vi "Drive Controller.vi"(8 "error in":errorcluster) -> ()   [LabVIEW 2017]
doc: "This VI executes continuously carrying out the current operation and responding to updates or new operation requests. It will often contain the timing or control code that is difficult to place directly in TeleOp. This VI generally opens all sensors and motors and isolates the rest of the robot code from knowing implementation details of how the operations are carried out."
uses:
  <vilib>/Rock Robotics/WPI/Framework/Completion Status.ctl
  Drive Setpoints.ctl
  Drive Operations.ctl
  Shared/RobotNeededPathData.ctl
  <vilib>/Rock Robotics/SystemInterfaces/DIO/FPGA_DIOPWMChannel.ctl
  <vilib>/Rock Robotics/WPI/SafetyOutput/WPI_SafetyOutputConfigMenu.ctl
  <vilib>/Rock Robotics/SystemInterfaces/DIO/FPGA_DIOChannel.ctl
  <vilib>/Rock Robotics/WPI/DriverStation/WPI_DriverStationRobotMode2.ctl
  <vilib>/Rock Robotics/WPI/RobotDrive/WPI_RobotDriveOpen2MotorWithSPARK.vi
  <vilib>/Rock Robotics/WPI/RobotDrive/WPI_RobotDriveOpen4MotorWithSPARK.vi
  <vilib>/Rock Robotics/WPI/Counter/WPI_CounterDigitalInputToDigitalSource.vi
  <vilib>/Rock Robotics/Network Tables/NT Read Number.vi
  Drive Published Globals.vi
  Framework/Robot Global Data.vi
  Configuration/Constants.vi
  <vilib>/Rock Robotics/WPI/ThirdParty/Sensors/navX/_Processing Loop/FRIC_navX_Internal_SPI_ProcessingLoop.vi
panel:
  in  "LookAhead":dbl=15.0 format="%#_13g"
  in  "Trackwidth":dbl=40.0 format="%#_13g"
  out "Yaw":dbl
  in  "Zero Yaw":bool
  in  "Gains":T1={"FFV"=0.0088, "FFA"=0.0017, "Vel PID"={"P"=0.01, "I"=0.007, "D"=0.0}}
  in  "Interactive Values":T2
  in  "Buttons":cluster{"Execute Cmd":bool, "Abort Cmd":bool}
  out "Command Timing":cluster{"Start Time (ms)":u32, "Iterations":i32}
  out "Status":T5
  out "Setpoints":T6(graph)
  out "Current\nCmd":string
  # "Tip: The graph shows the motor setpoints. It may also be helpful to observe inputs and sensor values.\nYou may also want to display tuning or debugging controls."
  # "Interactive Command: You may fill in the settings for a command\nand schedule it with the Execute button. You can observe and abort\nany command while fine tuning the code for the controller."
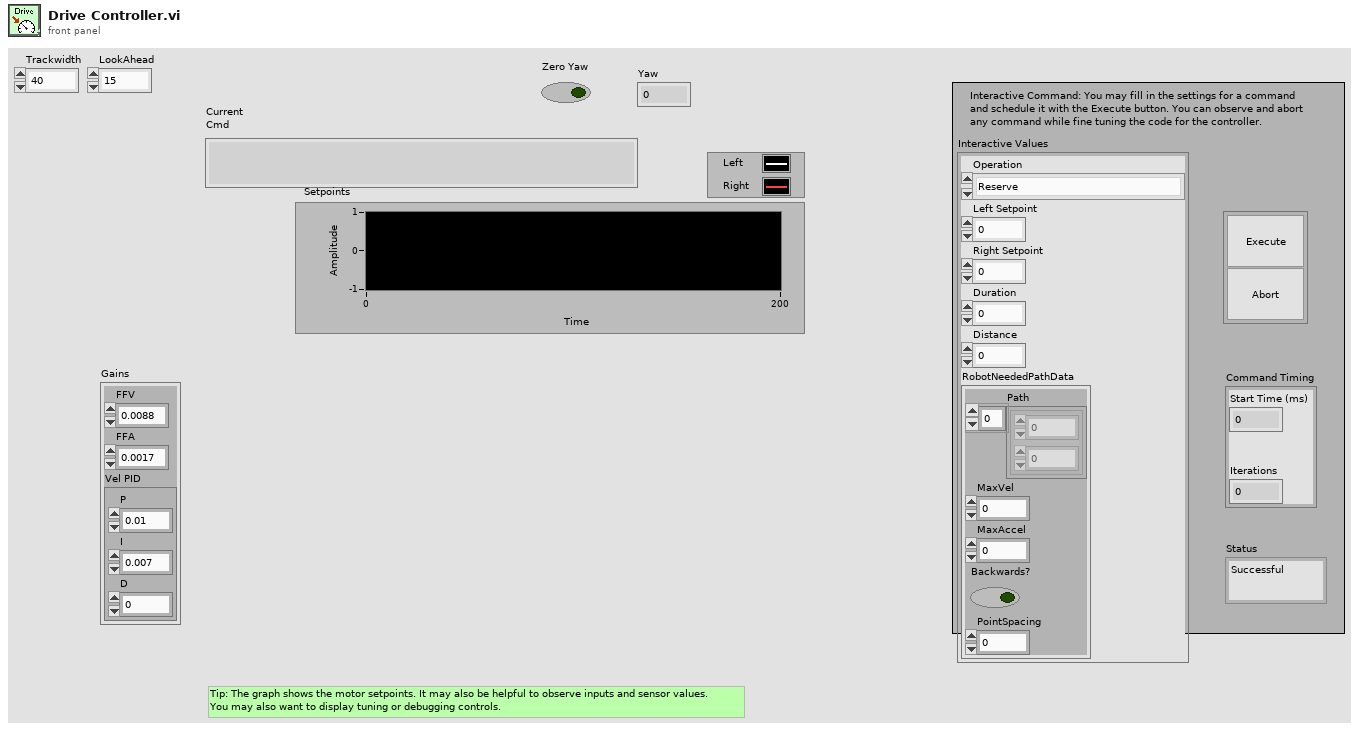
[diagram p1: front panel]
types:
  T1 = cluster{"FFV":dbl, "FFA":dbl, "Vel PID":cluster{"P":dbl, "I":dbl, "D":dbl}}
  T2 = typedef "Drive Setpoints.ctl" = cluster{"Operation":T3, "Left Setpoint":dbl, "Right Setpoint":dbl, "Duration":dbl, "Distance":dbl, "RobotNeededPathData":T4}
  T3 = typedef "Drive Operations.ctl" = enum16{"Reserve", "Read Current", "Immediate", "Drive for Time", "Drive for Distance", "Drive Path"}
  T4 = typedef "RobotNeededPathData.ctl" = cluster{"Path":cluster{dbl, dbl}[], "MaxVel":dbl, "MaxAccel":dbl, "Backwards?":bool, "PointSpacing":dbl}
  T5 = typedef "Completion Status.ctl" = enum16{"Successful", "Aborted", "Incomplete"}
  T6 = cluster{"Left Setpoint":dbl, "Right Setpoint":dbl}
  T7 = typedef "FPGA_DIOChannel.ctl" = enum8{"DIO 0", "DIO 1", "DIO 2", "DIO 3", "DIO 4", "DIO 5", "DIO 6", "DIO 7", "DIO 8", "DIO 9", "DIO MXP 0", "DIO MXP 1", "DIO MXP 2", "DIO MXP 3", "DIO MXP 4", "DIO MXP 5", "DIO MXP 6", "DIO MXP 7", "DIO MXP 8", "DIO MXP 9", "DIO MXP 10", "DIO MXP 11", "DIO MXP 12", "DIO MXP 13", "DIO MXP 14", "DIO MXP 15", "SPI Port CS1", "SPI Port CS2", "SPI Port CS3", "SPI Port MISO", "SPI Port MOSI", "Invalid"}
  T8 = typedef "WPI_SafetyOutputConfigMenu.ctl" = enum16{"Enable", "Disable"}
  T9 = typedef "FPGA_DIOPWMChannel.ctl" = enum8{"PWM 0", "PWM 1", "PWM 2", "PWM 3", "PWM 4", "PWM 5", "PWM 6", "PWM 7", "PWM 8", "PWM 9", "PWM MXP 0", "PWM MXP 1", "PWM MXP 2", "PWM MXP 3", "PWM MXP 4", "PWM MXP 5", "PWM MXP 6", "PWM MXP 7", "PWM MXP 8", "PWM MXP 9", "Invalid"}
  T10 = typedef "WPI_DigitalInputDevRef.ctl" = cluster{"DevStatus":errorcluster, "DIO Channel":T7}
  T11 = typedef "FPGA_CounterEncoderSourceConvertionLVSourceType.ctl" = cluster{"DevStatus":errorcluster, "AnalogTriggerMode?":bool, "DigitalMode":cluster{"DIO Channel":T12}, "AnalogTriggerMode":cluster{"AnalogTriggerIndex":T13, "OutputType":T14}}
  T12 = typedef "FPGA_DIODigitalSourceChannel.ctl" = enum8{"DIO 0", "DIO 1", "DIO 2", "DIO 3", "DIO 4", "DIO 5", "DIO 6", "DIO 7", "DIO 8", "DIO 9", "DIO MXP 0", "DIO MXP 1", "DIO MXP 2", "DIO MXP 3", "DIO MXP 4", "DIO MXP 5", "DIO MXP 6", "DIO MXP 7", "DIO MXP 8", "DIO MXP 9", "DIO MXP 10", "DIO MXP 11", "DIO MXP 12", "DIO MXP 13", "DIO MXP 14", "DIO MXP 15", "Disabled"}
  T13 = typedef "FPGA_AnalogTriggerIndex.ctl" = enum8{"Trig 0", "Trig 1", "Trig 2", "Trig 3", "Trig 4", "Trig 5", "Trig 6", "Trig 7", "Invalid"}
  T14 = typedef "FPGA_AnalogTriggerOutType.ctl" = enum16{"InWindow", "TriggerState", "Rising", "Falling"}
  T15 = typedef "WPI_EncoderDevRef.ctl" = cluster{"DevStatus":errorcluster, "EncoderIndex":T16, "CounterIndex":T17, "DistancePerCount":dbl, "Decoding Type":T18}
  T16 = typedef "FPGA_EncoderIdx.ctl" = enum8{"Enc 0", "Enc 1", "Enc 2", "Enc 3", "Enc 4", "Enc 5", "Enc 6", "Enc 7", "Invalid"}
  T17 = typedef "FPGA_CounterCtrSystemIndex.ctl" = enum8{"Ctr 0", "Ctr 1", "Ctr 2", "Ctr 3", "Ctr 4", "Ctr 5", "Ctr 6", "Ctr 7", "Invalid"}
  T18 = typedef "WPI_EncoderType.ctl" = enum16{"1x", "2x", "4x"}
  T19 = typedef "WPI_RobotDriveDevRef.ctl" = cluster{"DevStatus":errorcluster, "Motors[]":T20[], "Square Inputs":bool, "Max Output":dbl}
  T20 = typedef "WPI_MotorControlDeviceRef.ctl" = cluster{"DeviceStatus":errorcluster, "Type":T21, "PWM":cluster{"PWM Channel":T9, "DeadBand":T22}, "CAN":cluster{"Device Number":u8, "SetOutput VI Ref":variant, "GetOutput VI Ref":variant, "Enable VI Ref":variant, "Disable VI Ref":variant, "Data":variant}, "Invert":bool, "DIO PWM":cluster{"PWM \"Enable\" Channel":T9, "DIOChannel":T7, "PWM Rate":dbl}}
  T21 = typedef "WPI_MotorControlType.ctl" = enum16{"PWM", "CAN", "DIO PWM"}
  T22 = typedef "WPI_PWMDeadband.ctl" = cluster{"Name":string, "maxPositivePwm":i32, "minPositivePwm":i32, "centerPwm":i32, "maxNegativePwm":i32, "minNegativePwm":i32, "angularRange":u16}
  T23 = cluster{"RobotDriveDevRef":T19, "RobotDriveDevRef":T19}
  T24 = typedef "Command Status Info.ctl" = cluster{"Name":string, "Status":T5, "notifier out":T25}
  T25 = typedef "Completion Notifier.ctl" = refnum<notifier>
  T26 = cluster{"SubSystem Data":T2, cluster{"Start Time (ms)":u32, "Iterations":i32}, cluster{"Command Info":T24, "Description":string, "Default Command":T2, "queue out":refnum<queue>, "Subsystem Name":string}}
  T27 = cluster{"LeftDistance":dbl, "RightDistance":dbl, "LeftVelocity":dbl, "RightVelocity":dbl, "Angle":dbl, "Location":cluster{dbl, dbl}}
  T28 = cluster{"dx/dt":dbl, "dx/dt":dbl, "Yaw":dbl, cluster{dbl, dbl}}
  T29 = cluster{"Path":cluster{dbl, dbl}[], "PointSpacing":dbl}
  T30 = cluster{"SubSystem Data":T2, cluster{"Start Time (ms)":u32, "Iterations":i32}, "Default Command Arguments":cluster{"Command Info":T24, "Description":string, "Default Command":T2, "queue out":refnum<queue>, "Subsystem Name":string}}
  T31 = typedef "WPI_DriverStationRobotMode2.ctl" = enum16{"Autonomous Disabled", "Autonomous Enabled", "Teleop Disabled", "Teleop Enabled", "Disconnected", "Finish", "Test Disabled", "Test Enabled", "Emergency Stopped"}
  T32 = cluster{"Yaw":dbl, "Roll":dbl, "Pitch":dbl, "Heading":dbl, "Fused Heading":dbl}
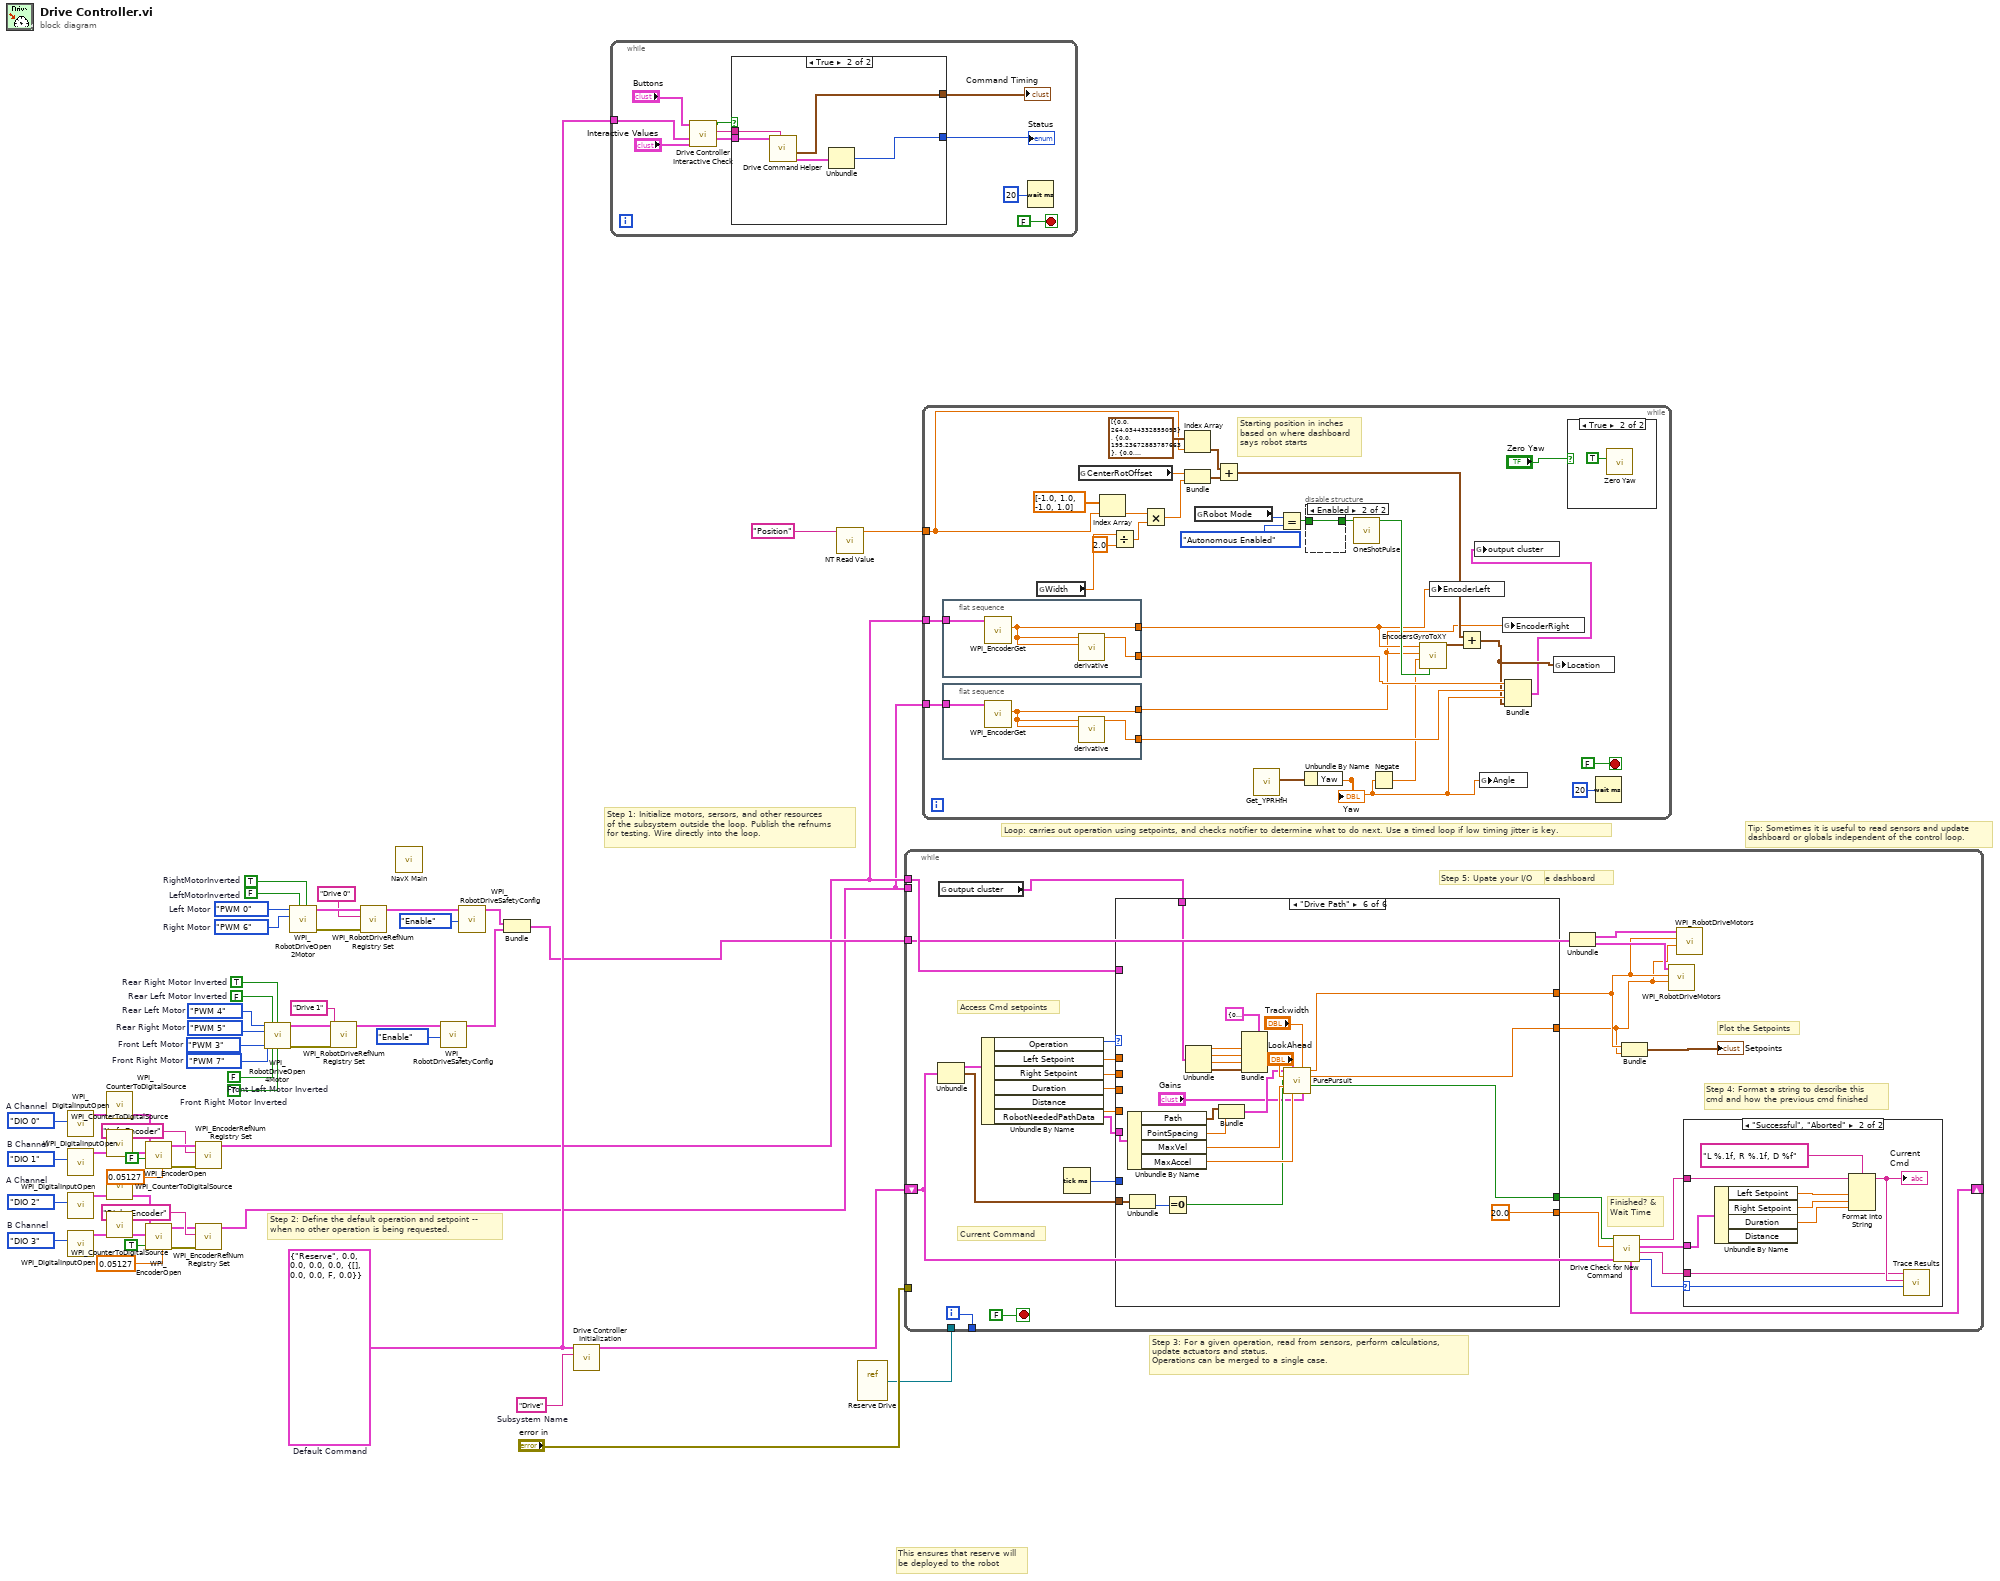
[diagram p0: block diagram]
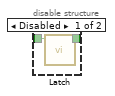
[diagram p2: hidden frame]
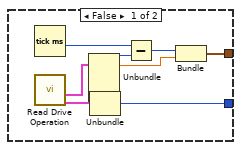
[diagram p4: hidden frame]
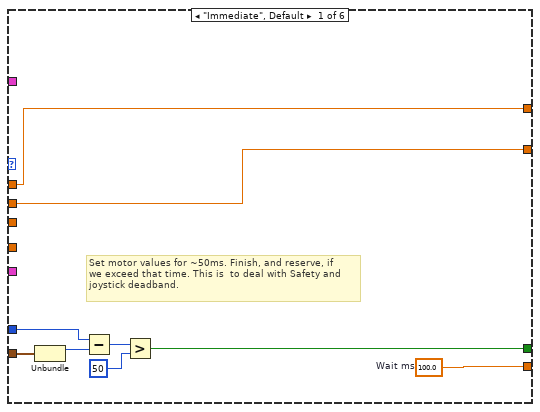
[diagram p5: hidden frame]
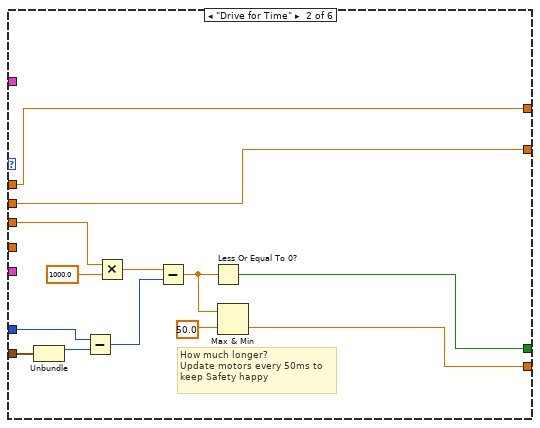
[diagram p6: hidden frame]
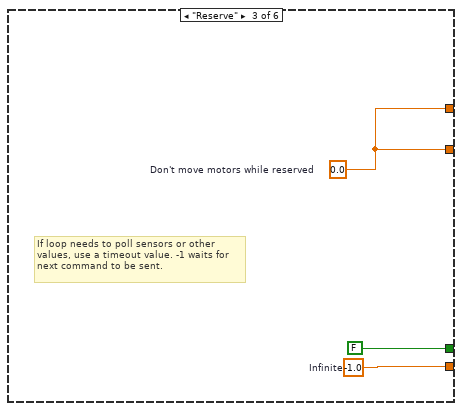
[diagram p7: hidden frame]
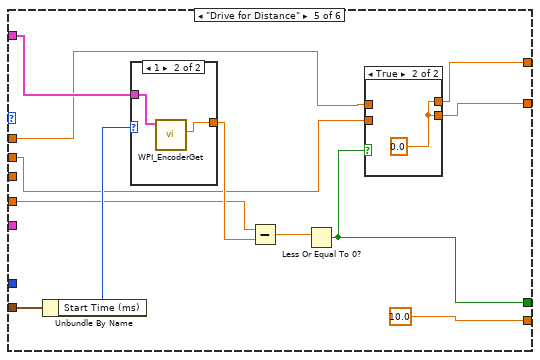
[diagram p9: hidden frame]
diagram:
  w9 = FPGA_DIOChannel."DIO 3"  # B Channel
  w10 = FPGA_DIOChannel."DIO 2"  # A Channel
  w26 = FPGA_DIOChannel."DIO 1"  # B Channel
  w25 = FPGA_DIOChannel."DIO 0"  # A Channel
  w32 = TRUE  # Front Right Motor Inverted
  w33 = FALSE  # Front Left Motor Inverted
  w34 = FALSE  # Rear Left Motor Inverted
  w35 = TRUE  # Rear Right Motor Inverted
  w38 = FPGA_DIOPWMChannel."PWM 7"  # Front Right Motor
  w39 = FPGA_DIOPWMChannel."PWM 3"  # Front Left Motor
  w40 = FPGA_DIOPWMChannel."PWM 5"  # Rear Right Motor
  w41 = FPGA_DIOPWMChannel."PWM 4"  # Rear Left Motor
  w46 = FPGA_DIOPWMChannel."PWM 6"  # Right Motor
  w47 = FPGA_DIOPWMChannel."PWM 0"  # Left Motor
  w50 = FALSE  # LeftMotorInverted
  w51 = TRUE  # RightMotorInverted
  w52 = T2 {"Operation"=enum."Reserve", "Left Setpoint"=0.0, "Right Setpoint"=0.0, "Duration"=0.0, "Distance"=0.0, "RobotNeededPathData"={"Path"=[], "MaxVel"=0.0, "MaxAccel"=0.0, "Backwards?"=FALSE, "PointSpacing"=0.0}}  # Default Command
  w56 = "Drive"  # Subsystem Name
  # "Step 3: For a given operation, read from sensors, perform calculations,\nupdate actuators and status.\nOperations can be merged to a single case."
  # "Step 2: Define the default operation and setpoint --\nwhen no other operation is being requested."
  # "This ensures that reserve will\nbe deployed to the robot"
  # "Tip: Sometimes it is useful to read sensors and update\ndashboard or globals independent of the control loop."
  # "Step 1: Initialize motors, sersors, and other resources\nof the subsystem outside the loop. Publish the refnums\nfor testing. Wire directly into the loop."
  # "Loop: carries out operation using setpoints, and checks notifier to determine what to do next. Use a timed loop if low timing jitter is key."
  n1 = call <vilib>:"WPI_DigitalInputOpen.vi"("DIO Channel"=w25) -> ("DigitalInputDevRef"=w22:T10)  [unwired: 1 in, 9 out]
  n2 = call <vilib>:"WPI_DigitalInputOpen.vi"("DIO Channel"=w26) -> ("DigitalInputDevRef"=w23:T10)  [unwired: 1 in, 9 out]
  n3 = call <vilib>:"WPI_DigitalInputOpen.vi"("DIO Channel"=w10) -> ("DigitalInputDevRef"=w13:T10)  [unwired: 1 in, 9 out]
  n4 = call <vilib>:"WPI_DigitalInputOpen.vi"("DIO Channel"=w9) -> ("DigitalInputDevRef"=w12:T10)  [unwired: 1 in, 9 out]
  n5 = call-poly <vilib>:"WPI_CounterToDigitalSource.vi"("DigitalInputDevRef"=w22) -> ("Digital Source"=w21:T11)  [unwired: 6 out]
  n6 = call-poly <vilib>:"WPI_CounterToDigitalSource.vi"("DigitalInputDevRef"=w23) -> ("Digital Source"=w24:T11)  [unwired: 6 out]
  n7 = call-poly <vilib>:"WPI_CounterToDigitalSource.vi"("DigitalInputDevRef"=w13) -> ("Digital Source"=w14:T11)  [unwired: 6 out]
  n8 = call-poly <vilib>:"WPI_CounterToDigitalSource.vi"("DigitalInputDevRef"=w12) -> ("Digital Source"=w11:T11)  [unwired: 6 out]
  n9 = call <vilib>:"WPI_EncoderOpen.vi"("DistancePerCount"=0.05127, "Invert Direction (False)"=FALSE, "BSource"=w24, "ASource"=w21) -> ("error out"=w20:errorcluster, "EncoderDevRef"=w19:T15)  [unwired: 4 in, 2 out]
  n10 = call <vilib>:"WPI_EncoderOpen.vi"("DistancePerCount"=0.05127, "Invert Direction (False)"=TRUE, "BSource"=w11, "ASource"=w14) -> ("error out"=w15:errorcluster, "EncoderDevRef"=w16:T15)  [unwired: 4 in, 2 out]
  n11 = call <vilib>:"WPI_EncoderRefNum Registry Set.vi"("error in (no error)"=w20, "refnum name"="Left Encoder", "EncoderDevRef"=w19) -> ("EncoderDevRef"=w4:T15)  [unwired: 7 in, 1 out]
  n12 = call <vilib>:"WPI_EncoderRefNum Registry Set.vi"("error in (no error)"=w15, "refnum name"="Right Encoder", "EncoderDevRef"=w16) -> ("EncoderDevRef"=w3:T15)  [unwired: 7 in, 1 out]
  n13 = call-poly <vilib>:"WPI_RobotDriveOpen4Motor.vi"("Rear Left Motor"=w41, "Rear Left Motor Inverted"=w34, "Rear Right Motor Inverted"=w35, "Rear Right Motor"=w40, "Front Left Motor"=w39, "Front Right Motor"=w38, "Front Left Motor Inverted"=w33, "Front Right Motor Inverted"=w32) -> ("RobotDriveDevRef"=w42:T19, "error out"=w43:errorcluster)  [unwired: 6 in]
  n14 = call-poly <vilib>:"WPI_RobotDriveOpen2Motor.vi"("Right Motor Inverted"=w51, "Left Motor Inverted"=w50, "Right Motor"=w46, "Left Motor"=w47) -> ("error out"=w48:errorcluster, "RobotDriveDevRef"=w49:T19)  [unwired: 1 in, 5 out]
  n15 = call <vilib>:"WPI_RobotDriveRefNum Registry Set.vi"("error in (no error)"=w43, "refnum name"="Drive 1", "RobotDriveDevRef"=w42) -> ("RobotDriveDevRef"=w37:T19)  [unwired: 7 in, 1 out]
  n16 = call <vilib>:"WPI_RobotDriveRefNum Registry Set.vi"("error in (no error)"=w48, "refnum name"="Drive 0", "RobotDriveDevRef"=w49) -> ("RobotDriveDevRef"=w45:T19)  [unwired: 1 in, 7 out]
  n17 = call-poly <vilib>:"NavX Main.vi"() -> ()  [unwired: 12 in]
  n18 = call <vilib>:"WPI_RobotDriveSafetyConfig.vi"("mode"=WPI_SafetyOutputConfigMenu."Enable", "RobotDriveDevRef"=w37) -> ("RobotDriveDevRef"=w28:T19)  [unwired: 8 in, 1 out]
  n19 = call <vilib>:"WPI_RobotDriveSafetyConfig.vi"("mode"=WPI_SafetyOutputConfigMenu."Enable", "RobotDriveDevRef"=w45) -> ("RobotDriveDevRef"=w29:T19)  [unwired: 8 in, 1 out]
  n20 = Bundle("RobotDriveDevRef"=w29, "RobotDriveDevRef"=w28) -> (w27:T23)  [unwired: 1 in]
  n21 = call "Drive Controller Initialization.vi"("Subsystem Name"=w56, "Default Command"=w52) -> ("Current Command"=w54:T26)  [unwired: 9 in]
  n22 = while {
    tunnel: w52 -> [w58]
    stop <- FALSE stop-if-true
    n23 = call "Drive Controller Interactive Check.vi"("Interactive Command In"="Interactive Values", "Default Command"=w58, "Buttons"="Buttons") -> ("Interactive Command Out"=w60:T2, "Trace String"=w61:string, "Schedule"=w62:bool)  [unwired: 6 in]
    n24 = case shown="True" w62 {
      tunnel: [w71 w79] -> w63
      tunnel: [w70 w75] -> w64
      tunnel: w61 -> [_ w77]
      tunnel: w60 -> [_ w76]
      frame False {
        n25 = Tick Count (ms)() -> (millisecond timer value=w74:u32)
        n26 = call "Read Drive Operation.vi"() -> ("Command Info"=w68:T24, "SubSystem Data"=w67:T2)  [unwired: 9 in, 1 out]
        n27 = Unbundle(w67) -> ("Operation"=w72:T3, "Left Setpoint"=w69:dbl)  [unwired: 4 out]
        n28 = Unbundle(w68) -> ("Status"=w71:T5)  [unwired: 2 out]
        n29 = Subtract(x=w74, y=w72) -> (x-y=w73:u32)
        n30 = Bundle(w73, "Left Setpoint"=w69) -> (w70:cluster{u32, "Left Setpoint":dbl})  [unwired: 1 in]
      }
      frame True {
        n31 = call "Drive Command Helper.vi"("Description"=w77, "SubSystem Data"=w76) -> ("Command Info Out"=w78:T24, "Command Timing"=w75:cluster{"Start Time (ms)":u32, "Iterations":i32})  [unwired: 7 in, 1 out]
        n32 = Unbundle(w78) -> ("Status"=w79:T5)  [unwired: 2 out]
      }
    }
    "Status" <- w63
    "Command Timing" <- w64
    n33 = Wait (ms)(milliseconds to wait=u32 20) -> ()  [unwired: 1 out]
  }
  n34 = call-poly <vilib>:"NT Read Value.vi"("Name"="Position") -> ("Numeric"=w1:dbl)  [unwired: 9 in, 1 out]
  n35 = vi-ref "Reserve Drive.vi"() -> (w53:refnum<vi>)
  n36 = while {
    shift-right: [w101] -> _
    shift-left: w54 -> [w96]
    tunnel: [w105] -> _
    tunnel: w27 -> [w85]
    tunnel: "error in" -> [_]
    tunnel: w53 -> [_]
    tunnel: w4 -> [w93]
    tunnel: w3 -> [_]
    i -> [w105]
    stop <- FALSE stop-if-true
    # "Step 5: Upate your I/O"
    # "Step 4: Format a string to describe this\ncmd and how the previous cmd finished"
    # "Current Command"
    # "Update motors and update dashboard"
    # "Plot the Setpoints"
    # "Access Cmd setpoints"
    # "Finished? &\nWait Time"
    n37 = Unbundle(w96) -> ("SubSystem Data"=w87:T2, w97:cluster{"Start Time (ms)":u32, "Iterations":i32})  [unwired: 1 out]
    n38 = global read "Drive Published Globals.vi" "output cluster"() -> (w80:T28)
    n39 = Unbundle By Name(w87) -> ("Operation"=w92:T3, "Left Setpoint"=w91:dbl, "Right Setpoint"=w90:dbl, "Duration"=w89:dbl, "Distance"=w88:dbl, "RobotNeededPathData"=w86:T4)
    n40 = Tick Count (ms)() -> (millisecond timer value=w103:u32)
    n41 = case shown="\"Drive Path\"" w92 {
      tunnel: w97 -> [w111 w125 _ _ w138 w160]
      tunnel: w91 -> [w109 w119 _ _ w134 _]
      tunnel: w90 -> [w108 w118 _ _ w135 _]
      tunnel: w89 -> [_ w123 _ _ _ _]
      tunnel: w103 -> [w112 w122 _ _ _ _]
      tunnel: [w110 w117 FALSE ("ignore previous (F)") _ w143 w167] -> w95
      tunnel: [w109 w119 w129 _ w133 w169] -> w82
      tunnel: [w108 w118 w129 _ w132 w168] -> w81
      tunnel: w93 -> [_ _ _ _ w140 _]
      tunnel: w88 -> [_ _ _ _ w137 _]
      tunnel: [w107 w116 w130 _ 10.0 ("Infinite") 20.0 ("Infinite")] -> w94
      tunnel: w86 -> [_ _ _ _ _ w165]
      tunnel: w80 -> [_ _ _ _ _ w151]
      frame "Immediate", Default {
        w107 = 100.0  # Wait ms
        # "Set motor values for ~50ms. Finish, and reserve, if\nwe exceed that time. This is  to deal with Safety and\njoystick deadband."
        n42 = Unbundle(w111) -> ("Start Time (ms)"=w113:u32)  [unwired: 1 out]
        n43 = Subtract(x=w112, y=w113) -> (x-y=w114:u32)
        n44 = Greater?(x=w114, y=u8 50 ("Left Motor")) -> (0:w110:bool)
      }
      frame "Drive for Time" {
        # "How much longer?\nUpdate motors every 50ms to\nkeep Safety happy"
        n45 = Unbundle(w125) -> ("Start Time (ms)"=w124:u32)  [unwired: 1 out]
        n46 = Subtract(x=w122, y=w124) -> (x-y=w128:u32)
        n47 = Multiply(x=w123, y=1000.0) -> (x*y=w127:dbl)
        n48 = Subtract(x=w127, y=w128) -> (x-y=w121:dbl)
        n49 = Less Or Equal To 0?(x=w121) -> (x <= 0?=w117:bool)
        n50 = Max & Min(x=w121, y=50.0) -> (min(x,y)=w116:dbl)  [unwired: 1 out]
      }
      frame "Reserve" {
        w129 = 0.0  # Don't move motors while reserved
        w130 = -1.0  # Infinite
        # "If loop needs to poll sensors or other\nvalues, use a timeout value. -1 waits for\nnext command to be sent."
      }
      frame "Read Current" {
      }
      frame "Drive for Distance" {
        n51 = Unbundle By Name(w138) -> ("Start Time (ms)"=w139:u32)
        n52 = case shown="1" w139 {
          tunnel: w140 -> [_ w145]
          tunnel: [_ w144] -> w141
          frame 0, Default {
          }
          frame 1 {
            n53 = call <vilib>:"WPI_EncoderGet.vi"("EncoderDevRef"=w145) -> ("Distance"=w144:dbl)  [unwired: 5 in, 5 out]
          }
        }
        n54 = Subtract(x=w137, y=w141) -> (x-y=w142:dbl)
        n55 = Less Or Equal To 0?(x=w142) -> (x <= 0?=w143:bool)
        n56 = case shown="True" w143 {
          tunnel: [_ w146] -> w132
          tunnel: w134 -> [_ _]
          tunnel: w135 -> [_ _]
          tunnel: [_ w146] -> w133
          frame False {
          }
          frame True {
            w146 = 0.0
          }
        }
      }
      frame "Drive Path" {
        n57 = Unbundle By Name(w165) -> ("Path"=w159:cluster{dbl, dbl}[], "PointSpacing"=w158:dbl, "MaxVel"=w156:dbl, "MaxAccel"=w155:dbl)
        n58 = Unbundle(w160) -> ("Iterations"=w154:i32)  [unwired: 1 out]
        n59 = Equal To 0?(x=w154) -> (x = 0?=w153:bool)
        n60 = Unbundle(w151) -> ("dx/dt"=w150:dbl, "dx/dt"=w149:dbl, "Yaw"=w148:dbl, w147:cluster{dbl, dbl})
        n61 = Bundle("Path"=w159, "PointSpacing"=w158) -> (w157:T29)  [unwired: 1 in]
        n62 = Bundle(cluster=T27 {"LeftDistance"=0.0, "RightDistance"=0.0, "LeftVelocity"=0.0, "RightVelocity"=0.0, "Angle"=0.0, "Location"={0.0, 0.0}} ("SensorData"), "LeftVelocity"=w150, "RightVelocity"=w149, "Angle"=w148, "Location"=w147) -> (w164:T27)  [unwired: 2 in]
        n63 = call "PurePursuit.vi"("PathData"=w157, "SensorData"=w164, "Trackwidth"="Trackwidth", "LookAhead"="LookAhead", "Reset"=w153, "MaxVel"=w156, "Max Accel"=w155, "Gains"="Gains") -> ("LeftValue"=w169:dbl, "RightValue"=w168:dbl, "Done"=w167:bool)  [unwired: 3 in, 2 out]
      }
    }
    n64 = Unbundle(w85) -> ("RobotDriveDevRef"=w84:T19, "RobotDriveDevRef"=w83:T19)
    n65 = call "Drive Check for New Command.vi"("input cluster"=w96, "Wait time (ms)"=w94, "Finished?"=w95) -> ("Completion"=w102:T5, "Subsystem Name"=w98:string, "Current Command"=w99:T2, "Initial Trace String"=w100:string, "Next Command"=w101:T30)  [unwired: 4 in]
    n66 = Bundle("LeftValue"=w82, "RightValue"=w81) -> (→"Setpoints":cluster{"LeftValue":dbl, "RightValue":dbl})  [unwired: 1 in]
    n67 = call <vilib>:"WPI_RobotDriveMotors.vi"("RightSpeed"=w81, "LeftSpeed"=w82, "RobotDriveDevRef"=w83) -> ()  [unwired: 1 in, 8 out]
    n68 = call <vilib>:"WPI_RobotDriveMotors.vi"("RightSpeed"=w81, "LeftSpeed"=w82, "RobotDriveDevRef"=w84) -> ()  [unwired: 1 in, 8 out]
    n69 = case shown="\"Successful\", \"Aborted\"" w102 {
      selector: w102 -> [_ w178]
      tunnel: w100 -> [_ w176]
      tunnel: w99 -> [_ w173]
      tunnel: w98 -> [_ w174]
      frame "Incomplete", Default {
        # "Continuing current command"
      }
      frame "Successful", "Aborted" {
        # "Report and setup for next command"
        n70 = Unbundle By Name(w173) -> ("Left Setpoint"=w172:dbl, "Right Setpoint"=w171:dbl, "Duration"=w170:dbl)  [unwired: 1 out]
        n71 = Format Into String(format string="L %.1f, R %.1f, D %f", initial string=w176, w172, w171, w170) -> (resulting string=w175:string)  [unwired: 1 in, 1 out]
        "Current\nCmd" <- w175
        n72 = call <vilib>:"Trace Results.vi"("Status of previous command"=w178, "Description"=w175, "Subsystem"=w174) -> ()  [unwired: 9 in]
      }
    }
  }
  n73 = while {
    tunnel: w4 -> [w208]
    tunnel: w3 -> [w207]
    tunnel: w1 -> [w180]
    stop <- FALSE stop-if-true
    # "Starting position in inches\nbased on where dashboard\nsays robot starts"
    n74 = flat-sequence {
      tunnel: [w217] -> w188
      tunnel: [w216] -> w184
      tunnel: w208 -> [w215]
      frame #0 {
        n75 = call <vilib>:"WPI_EncoderGet.vi"("EncoderDevRef"=w215) -> ("Distance"=w216:dbl)  [unwired: 5 in, 5 out]
        n76 = call "derivative.vi"("Starting value"=w216, "x"=w216) -> ("dx/dt"=w217:dbl)  [unwired: 9 in]
      }
    }
    n77 = flat-sequence {
      tunnel: w207 -> [w218]
      tunnel: [w220] -> w187
      tunnel: [w219] -> w183
      frame #0 {
        n78 = call <vilib>:"WPI_EncoderGet.vi"("EncoderDevRef"=w218) -> ("Distance"=w219:dbl)  [unwired: 5 in, 5 out]
        n79 = call "derivative.vi"("Starting value"=w219, "x"=w219) -> ("dx/dt"=w220:dbl)  [unwired: 9 in]
      }
    }
    n80 = global read "Constants.vi" "Width"() -> (w202:dbl)
    n81 = global read "Constants.vi" "CenterRotOffset"() -> (w200:dbl)
    n82 = Index Array(array=dbl[] [-1.0, 1.0, -1.0, 1.0], index=w180) -> (element=w201:dbl)
    n83 = Divide(x=w202, y=2.0) -> (x/y=w196:dbl)
    n84 = Multiply(x=w201, y=w196) -> (x*y=w197:dbl)
    n85 = Index Array(array=cluster{dbl, dbl}[] [{0.0, 264.0344332855093}, {0.0, 195.23672883787663}, {0.0, 144.10329985652797}, {0.0, -0.0}] ("x*y"), index=w180) -> (element=w199:cluster{dbl, dbl})
    n86 = Bundle("CenterRotOffset"=w200, w197) -> (w198:cluster{"CenterRotOffset":dbl, dbl})  [unwired: 1 in]
    n87 = global read "Robot Global Data.vi" "Robot Mode"() -> (w205:T31)
    n88 = Add(x=w199, y=w198) -> (x+y=w189:cluster{dbl, dbl})
    n89 = call <vilib>:"Get_YPRHfH.vi"() -> ("YRPHfH"=w209:T32)  [unwired: 11 in]
    n90 = Equal?(x=w205, y=WPI_DriverStationRobotMode2."Autonomous Enabled") -> (x = y?=w203:bool)
    n91 = Unbundle By Name(w209) -> ("Yaw"=w182:dbl)
    "Yaw" <- w182
    n92 = disable-structure shown="Enabled" {
      disable-tunnel: w203 -> [w212 w213]
      disable-tunnel: [w211 w213] -> w192
      frame Disabled {
        n93 = call "Latch.vi"("Input"=w212) -> ("Output"=w211:bool)  [unwired: 10 in]
      }
      frame Enabled {
      }
    }
    n94 = call "OneShotPulse.vi"("Input"=w192) -> ("Output"=w191:bool)  [unwired: 10 in]
    n95 = Negate(x=w182) -> (-x=w186:dbl)
    n96 = call "EncodersGyroToXY.vi"("Reset"=w191, "Angle (degrees)"=w186, "Right Distance"=w183, "Left Distance"=w184) -> ("Location"=w190:cluster{dbl, dbl})  [unwired: 7 in]
    n97 = global write "Drive Published Globals.vi" "EncoderLeft"(w184) -> ()
    n98 = Add(x=w189, y=w190) -> (x+y=w181:cluster{dbl, dbl})
    n99 = global write "Drive Published Globals.vi" "Angle"(w182) -> ()
    n100 = global write "Drive Published Globals.vi" "EncoderRight"(w183) -> ()
    n101 = Bundle("dx/dt"=w188, "dx/dt"=w187, "Yaw"=w182, w181) -> (w179:T28)  [unwired: 1 in]
    n102 = global write "Drive Published Globals.vi" "output cluster"(w179) -> ()
    n103 = global write "Drive Published Globals.vi" "Location"(w181) -> ()
    n104 = case shown="True" "Zero Yaw" {
      frame False {
      }
      frame True {
        n105 = call <vilib>:"Zero Yaw.vi"("Zero"=TRUE) -> ()  [unwired: 11 in]
      }
    }
    n106 = Wait (ms)(milliseconds to wait=u32 20) -> ()  [unwired: 1 out]
  }
